vi "Arduino example 1.vi"() -> ()   [LabVIEW 2015]
uses:
  <vilib>/LabVIEW Interface for Arduino/LabVIEW Interface for Arduino.lvlib
panel:
  in  "STOP":bool
  out "Voltage":dbl(knob) scale=0.0..5.0
  in  "Analog Input Pin (0)":u8
  in  "VISA resource":refnum<visa-resource-name>
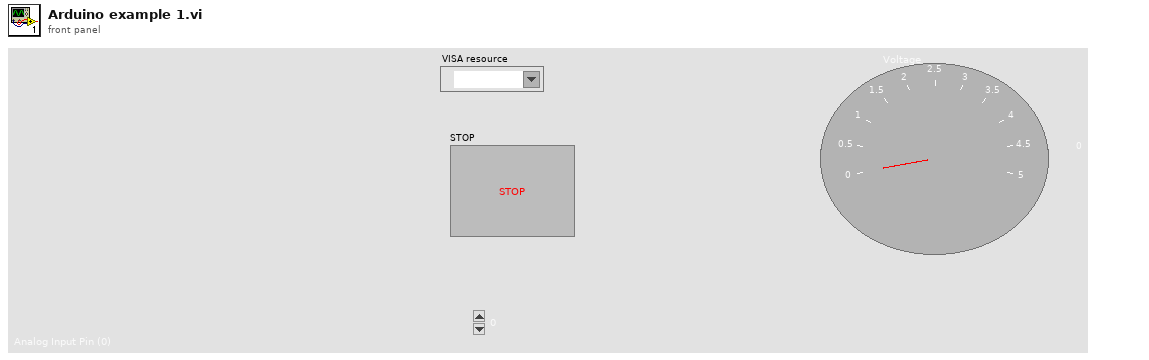
[diagram p1: front panel]
types:
  T1 = typedef "LabVIEW Interface for Arduino.lvlib/Arduino Resource.ctl" = cluster{"VISA resource":refnum<visa-resource-name>, "Board Type":T2, "Connection Type":enum8{"USB / Serial"}, "Bytes Per Packet (15)":u8}
  T2 = typedef "LabVIEW Interface for Arduino.lvlib/Board Type.ctl" = enum16{"Uno", "Dimuelanove w/Atmega 328", "Mega 2560"}
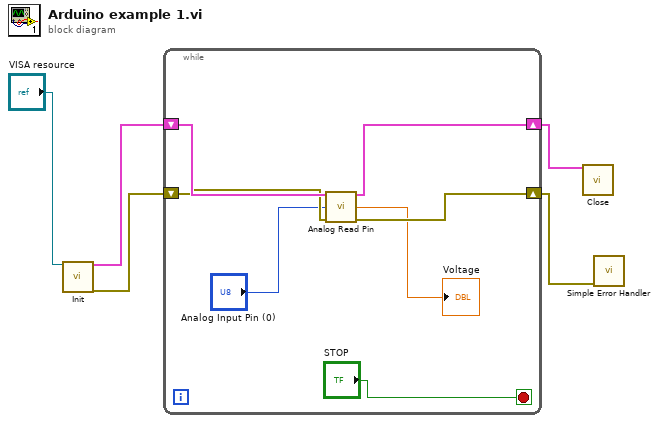
[diagram p0: block diagram]
diagram:
  n1 = call <vilib>:"Init.vi"("VISA resource"="VISA resource") -> ("Arduino Resource"=w5:T1, "error out"=w4:errorcluster)  [unwired: 17 in]
  n2 = while {
    shift-right: [w11] -> w2
    shift-left: w5 -> [w12]
    shift-right: [w9] -> w1
    shift-left: w4 -> [w10]
    stop <- "STOP" stop-if-true
    n3 = call <vilib>:"Analog Read Pin.vi"("Arduino Resource"=w12, "Analog Input Pin (0)"="Analog Input Pin (0)", "error in"=w10) -> ("Arduino Resource"=w11:T1, "Voltage"=→"Voltage":dbl, "error out"=w9:errorcluster)  [unwired: 10 in]
  }
  n4 = call <vilib>:"Close.vi"("Arduino Resource"=w2) -> ()  [unwired: 14 in, 1 out]
  n5 = call <vilib>:"Simple Error Handler.vi"("error in (no error)"=w1) -> ()  [unwired: 4 in, 5 out]
